vi "Read position -- subVI.vi"(8 "error in (no error)":errorcluster, 11 "VISA Refnum in":refnum<visa-resource-name>) -> (0 "error out":errorcluster, 3 "Current position":dbl)   [LabVIEW 2020, in "Monochromator.lvlib"]
uses:
  Monochromator.lvlib
  <vilib>/regexp/Match Regular Expression.xnode
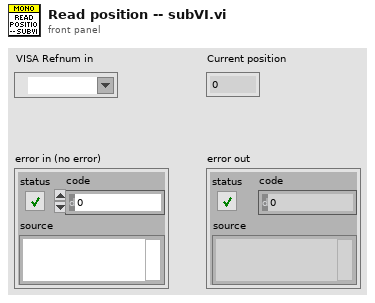
[diagram p1: front panel]
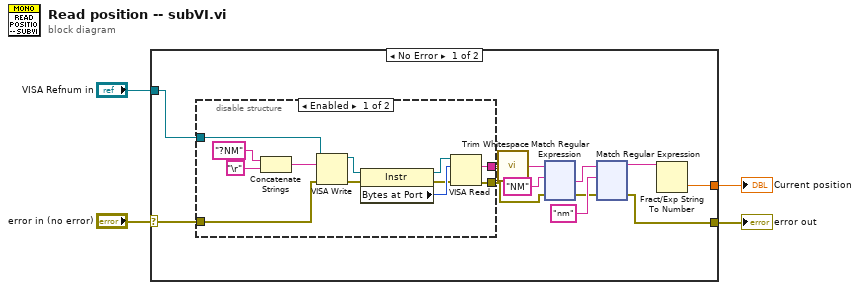
[diagram p0: block diagram]
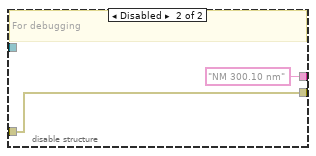
[diagram p2: hidden frame]
diagram:
  n1 = case shown="No Error" "error in (no error)" {
    selector: "error in (no error)" -> [w10 w259]
    tunnel: "VISA Refnum in" -> [w11 _]
    tunnel: [w6 w259] -> w2
    tunnel: [w5 _] -> w1
    frame No Error {
      n2 = disable-structure shown="Enabled" {
        disable-tunnel: [w28 "NM 300.10 nm" ("string")] -> w13
        disable-tunnel: w11 -> [w19 _]
        disable-tunnel: w10 -> [w18 w29]
        disable-tunnel: [w17 w29] -> w8
        frame Enabled {
          n3 = Concatenate Strings("?NM" ("string"), "\r") -> (w20:string)
          n4 = VISA Write(VISA resource name=w19, write buffer=w20, error in (no error)=w18) -> (VISA resource name out=w25:refnum<visa-resource-name>, error out=w23:errorcluster)  [unwired: 1 out]
          n5 = property class="Instr"(reference=w25, error in=w23) -> (reference out=w27:refnum<visa-resource-name>, error out=w24:errorcluster, "Bytes at Port"=w26:u32)
          n6 = VISA Read(VISA resource name=w27, byte count=w26, error in (no error)=w24) -> (read buffer=w28:string, error out=w17:errorcluster)  [unwired: 2 out]
        }
        frame Disabled {
          # "For debugging"
        }
      }
      n7 = call <vilib>:"Trim Whitespace.vi"("string"=w13) -> ("trimmed string"=w14:string)  [unwired: 1 in]
      n8 = xnode "Match Regular Expression"("input string"=w14, "regular expression"="NM", "error in"=w8) -> ("after match"=w15:string, "error out"=w7:errorcluster)  [unwired: 3 in, 3 out]
      n9 = xnode "Match Regular Expression"("input string"=w15, "regular expression"="nm", "error in"=w7) -> ("before match"=w9:string, "error out"=w6:errorcluster)  [unwired: 3 in, 3 out]
      n10 = Fract/Exp String To Number(string=w9) -> (number=w5:dbl)  [unwired: 3 in, 1 out]
    }
    frame Error {
    }
  }
  "error out" <- w2
  "Current position" <- w1
